vi "Initialize Repository.vi"(7 "config folder":path, 8 "error in (no error)":errorcluster, 11 "Path":path) -> (0 "error out":errorcluster, 2 "Files Copied":path[](array[path]))   [LabVIEW 2019, in "Build.lvlib"]
uses:
  Build.lvlib
  Git/Git.lvclass
  <vilib>/Utility/sysdir.llb/System Directory Type.ctl
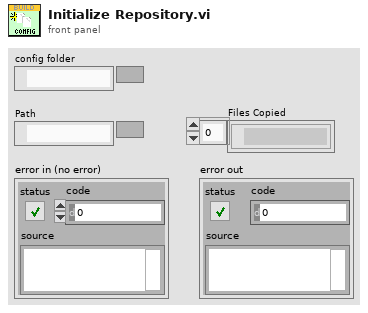
[diagram p1: front panel]
types:
  T1 = typedef "System Directory Type.ctl" = i32
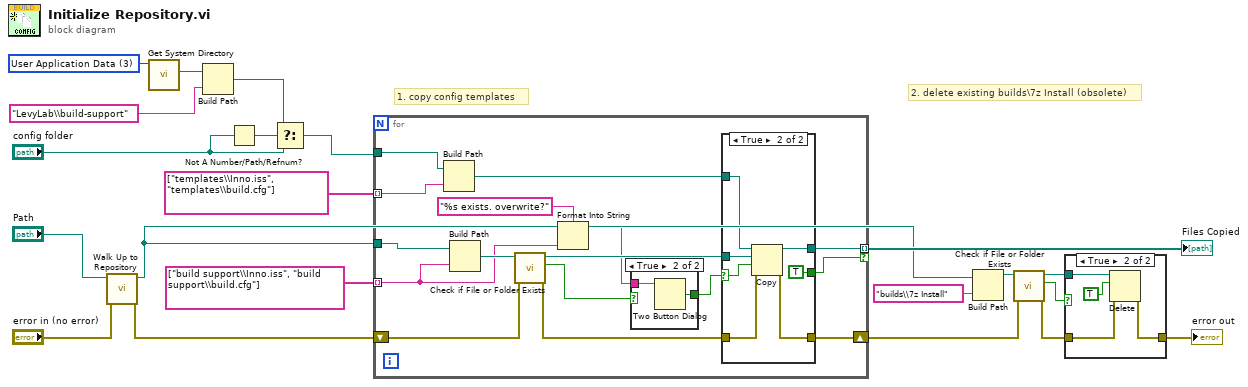
[diagram p0: block diagram]
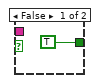
[diagram p2: hidden frame]
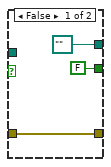
[diagram p3: hidden frame]
diagram:
  w7 = T1 3 items=["User Home"=0, "User Desktop"=1, "User Documents"=2, "User Application Data"=3, "User Preferences"=4, "User Temporary"=5, "Public Documents"=6, "Public Application Data"=7, "Public Preferences"=8, "Public Cache"=13, "System Core Libraries"=9, "System Installed Libraries"=10, "Application Files"=11, "Boot Volume Root"=12] ("system directory type")
  # "2. delete existing builds\\7z Install (obsolete)"
  # "1. copy config templates"
  n1 = call "Walk Up to Repository.vi"("error in (no error)"="error in (no error)", "Build Path"="Path") -> ("error out"=w18:errorcluster, "Repository Path"=w15:path)  [unwired: 8 in]
  n2 = call <vilib>:"Get System Directory.vi"("system directory type"=w7) -> ("system directory"=w6:path)  [unwired: 10 in]
  n3 = Build Path(base path=w6, name or relative path="LevyLab\\build-support") -> (appended path=w3:path)
  n4 = Not A Number/Path/Refnum?(number/path/refnum="config folder") -> (NaN/Path/Refnum?=w4:bool)
  n5 = Select(t=w3, s=w4, f="config folder") -> (s? t:f=w2:path)
  n6 = for {
    tunnel: string[] ["build support\\Inno.iss", "build support\\build.cfg"] ("name or relative path") -> [w22] mode=indexing
    tunnel: string[] ["templates\\Inno.iss", "templates\\build.cfg"] ("name or relative path") -> [w37] mode=indexing
    tunnel: w2 -> [w36]
    tunnel: w15 -> [w33]
    shift-right: [w32] -> w10
    shift-left: w18 -> [w35]
    tunnel: [w24] -> w16 mode=indexing if=w23
    n7 = Build Path(base path=w36, name or relative path=w37) -> (appended path=w29:path)
    n8 = Build Path(base path=w33, name or relative path=w22) -> (appended path=w31:path)
    n9 = call <vilib>:"Check if File or Folder Exists.vi"("error in (no error)"=w35, "path"=w31) -> ("error out"=w34:errorcluster, "file or folder exists?"=w28:bool, "dup path"=w30:path)  [unwired: 7 in]
    n10 = Format Into String(format string="%s exists. overwrite?", w22) -> (resulting string=w25:string)  [unwired: 2 in, 1 out]
    n11 = case shown="True" w28 {
      tunnel: [TRUE w40] -> w27
      tunnel: w25 -> [_ w39]
      frame False {
      }
      frame True {
        n12 = Two Button Dialog(message=w39) -> (T button?=w40:bool)  [unwired: 2 in]
      }
    }
    n13 = case shown="True" w27 {
      selector: w27 -> [_ w46]
      tunnel: w34 -> [w43 w50]
      tunnel: [w43 w49] -> w32
      tunnel: w30 -> [_ w48]
      tunnel: w29 -> [_ w47]
      tunnel: [path "" ("new path") w45] -> w24
      tunnel: [FALSE TRUE] -> w23
      frame False {
      }
      frame True {
        n14 = Copy(8:w50, 9:w46, 10:w48, 11:w47) -> (0:w49:errorcluster, 3:w45:path)  [unwired: 1 in, 1 out]
      }
    }
  }
  "Files Copied" <- w16
  n15 = Build Path(base path=w15, name or relative path="builds\\7z Install") -> (appended path=w12:path)
  n16 = call <vilib>:"Check if File or Folder Exists.vi"("error in (no error)"=w10, "path"=w12) -> ("error out"=w9:errorcluster, "file or folder exists?"=w8:bool, "dup path"=w11:path)  [unwired: 7 in]
  n17 = case shown="True" w8 {
    tunnel: [w51 w55] -> w13
    tunnel: w11 -> [_ w53]
    tunnel: w9 -> [w51 w52]
    frame False {
    }
    frame True {
      n18 = Delete(path (use dialog)=w53, entire hierarchy (F)=TRUE, error in=w52) -> (error out=w55:errorcluster)  [unwired: 2 in, 2 out]
    }
  }
  "error out" <- w13
